vi "Variant to Data.vi"(11 "Variant":variant) -> (0 "error out":errorcluster, 1 "String Value":string, 2 "Type":string, 3 "Value":string)   [LabVIEW 2020, in "CAML.lvlib" / "CAML.lvclass"]
uses:
  <vilib>/gpm_packages/@cs/persistence/source/CAML/CAML.lvclass
  <vilib>/gpm_packages/@cs/data-type-serializer/source/Data Type/Data Type.lvclass
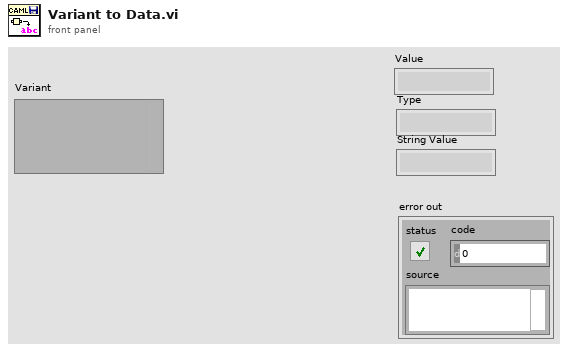
[diagram p1: front panel]
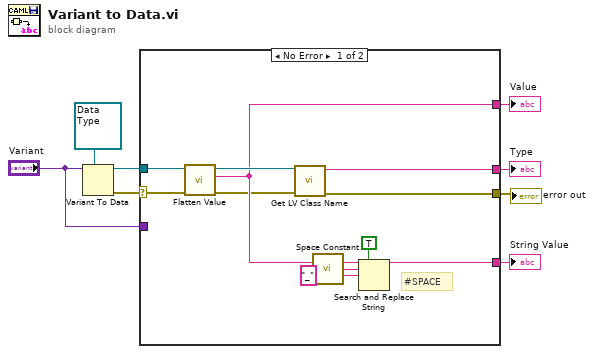
[diagram p0: block diagram]
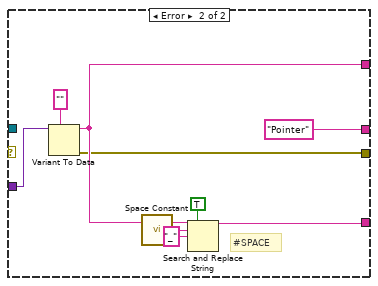
[diagram p2: hidden frame]
diagram:
  n1 = Variant To Data(type=refnum<class "Data Type.lvclass"> refnum ("Data Type.lvclass"), Variant="Variant") -> (data=w7:refnum<class "Data Type.lvclass">, error out=w6:errorcluster)  [unwired: 1 in]
  n2 = case shown="No Error" w6 {
    selector: w6 -> [w11 _]
    tunnel: w7 -> [w16 _]
    tunnel: "Variant" -> [_ w28]
    tunnel: [w14 w22] -> w4
    tunnel: [w13 "Pointer" ("class name")] -> w3
    tunnel: [w12 w24] -> w2
    tunnel: [w9 w20] -> w1
    frame No Error {
      # "#SPACE"
      n3 = call-dynamic "Flatten Value.vi"("error in (no error)"=w11, "Data Type in"=w16) -> ("error out"=w10:errorcluster, "Value"=w14:string, "Data Type out"=w15:refnum<class "Data Type.lvclass">)  [unwired: 7 in]
      n4 = call <vilib>:"Get LV Class Name.vi"("error in (no error)"=w10, "object"=w15) -> ("error out"=w9:errorcluster, "class name"=w13:string)  [unwired: 8 in]
      n5 = call <vilib>:"Space Constant.vi"() -> ("String"=w19:string)
      n6 = Search and Replace String(replace all?=TRUE ("replace all? (F)"), input string=w14, search string=w19, replace string="_") -> (result string=w12:string)  [unwired: 4 in, 3 out]
    }
    frame Error {
      # "#SPACE"
      n7 = Variant To Data(type="", Variant=w28) -> (data=w22:string, error out=w20:errorcluster)  [unwired: 1 in]
      n8 = call <vilib>:"Space Constant.vi"() -> ("String"=w26:string)
      n9 = Search and Replace String(replace all?=TRUE ("replace all? (F)"), input string=w22, search string=w26, replace string="_" ("replace string (\"\")")) -> (result string=w24:string)  [unwired: 4 in, 3 out]
    }
  }
  "Value" <- w4
  "Type" <- w3
  "String Value" <- w2
  "error out" <- w1
